vi "Configure Level.vi"(8 "Error In":errorcluster, 11 "Level":u8=7) -> (0 "Error Out":errorcluster)   [LabVIEW 2015, in "Logger.lvlib"]
doc: "Sets the global level for all listeners."
uses:
  Logger.lvlib
  Private/Action.ctl
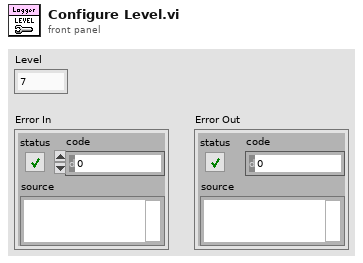
[diagram p1: front panel]
types:
  T1 = typedef "Logger.lvlib/Action.ctl" = enum16{"Initialize", "Register", "Log", "Unregister", "Set Level", "Shutdown"}
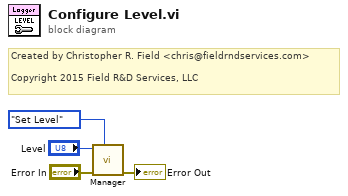
[diagram p0: block diagram]
diagram:
  # "Created by Christopher R. Field <chris@fieldrndservices.com>\n\nCopyright 2015 Field R&D Services, LLC"
  n1 = call "Manager.vi"("Action"=Action."Set Level", "Error In"="Error In", "Value In"="Level") -> ("Error Out"=→"Error Out":errorcluster)  [unwired: 8 in]
